vi "Calculate Line Reciprocal.vi"(10 "P2":T1, 11 "P1":T1) -> (3 "Column Pixels Per Row":sgl)   [LabVIEW 2020, in "Raster (FPGA).lvlib"]
uses:
  Raster (FPGA).lvlib
  3D/Vector 3D.ctl
  3D/3D (FPGA).lvlib
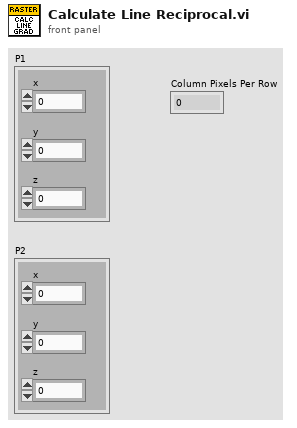
[diagram p1: front panel]
types:
  T1 = typedef "3D (FPGA).lvlib/Vector 3D.ctl" = cluster{"x":sgl, "y":sgl, "z":sgl}
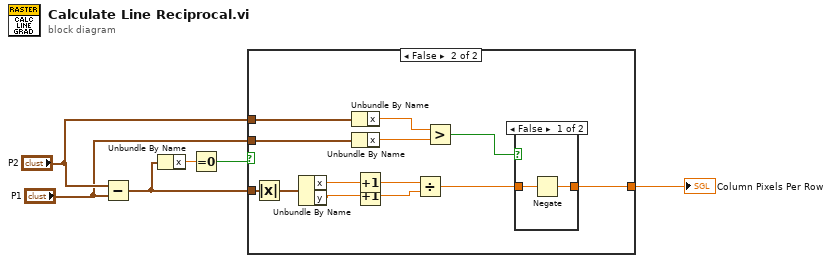
[diagram p0: block diagram]
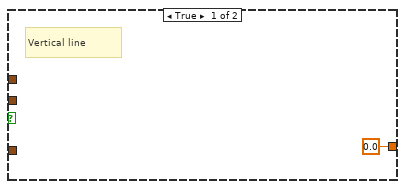
[diagram p2: hidden frame]
diagram:
  n1 = Subtract(x="P2", y="P1") -> (x-y=w3:T1)
  n2 = Unbundle By Name(w3) -> ("x"=w2:sgl)
  n3 = Equal To 0?(x=w2) -> (x = 0?=w1:bool)
  n4 = case shown="False" w1 {
    tunnel: w3 -> [_ w20]
    tunnel: "P2" -> [_ w14]
    tunnel: "P1" -> [_ w13]
    tunnel: [sgl 0.0 w8] -> w4
    frame True {
      # "Vertical line"
    }
    frame False {
      n5 = Absolute Value(x=w20) -> (abs(x)=w15:T1)
      n6 = Unbundle By Name(w15) -> ("x"=w19:sgl, "y"=w18:sgl)
      n7 = Unbundle By Name(w14) -> ("x"=w12:sgl)
      n8 = Unbundle By Name(w13) -> ("x"=w11:sgl)
      n9 = Increment(x=w19) -> (x+1=w17:sgl)
      n10 = Increment(x=w18) -> (x+1=w16:sgl)
      n11 = Divide(x=w17, y=w16) -> (x/y=w9:sgl)
      n12 = Greater?(x=w12, y=w11) -> (0:w10:bool)
      n13 = case shown="False" w10 {
        tunnel: w9 -> [w22 w23]
        tunnel: [w21 w23] -> w8
        frame False {
          n14 = Negate(x=w22) -> (-x=w21:sgl)
        }
        frame True {
        }
      }
    }
  }
  "Column Pixels Per Row" <- w4
